vi "clearTxBuffer.vi"(8 "error in (no error)":errorcluster, 11 "Modbus in":refnum<class "Modbus.lvclass">) -> (0 "error out":errorcluster, 3 "Modbus out":refnum<class "Modbus.lvclass">)   [LabVIEW 2015, in "Modbus.lvclass"]
uses:
  Modbus.lvclass
  Typedefs/Frame.ctl
  Modbus.lvclass/Modbus.ctl
  Typedefs/RTTypeDefs.lvlib
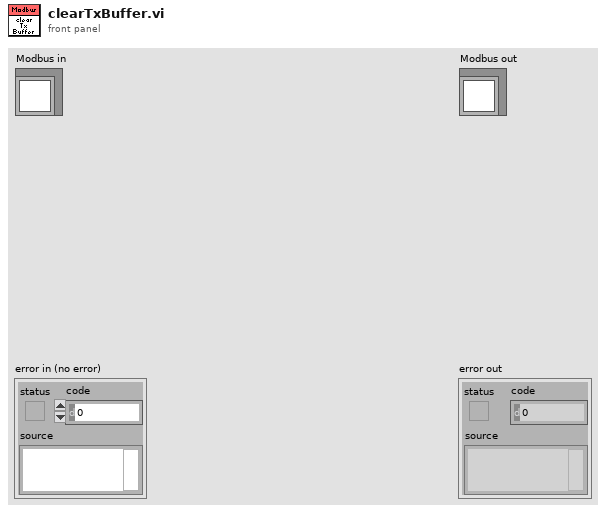
[diagram p1: front panel]
types:
  T1 = typedef "RTTypeDefs.lvlib/Frame.ctl" = cluster{"Data":u8[], "WaitForTrigger":bool, "WaitForRx":u16, "TriggerIRQ":i16}
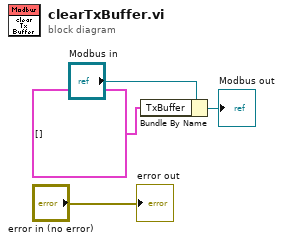
[diagram p0: block diagram]
diagram:
  n1 = Bundle By Name(cluster="Modbus in", "TxBuffer"=T1[] []) -> (→"Modbus out":refnum<class "Modbus.lvclass">)
  "error out" <- "error in (no error)"
